vi "Main.vi"() -> ()   [LabVIEW 2012]
uses:
  TypeDefs/States.ctl
  <vilib>/Analysis/NI_AALBase.lvlib
  <vilib>/Analysis/1siggen.llb/Ramp Pattern by Samples.vi
  <vilib>/DAQmx/write.llb/DAQmx Write (Digital Bool 1Line 1Point).vi
  <vilib>/DAQmx/write.llb/DAQmx Write (Analog 1D DBL NChan 1Samp).vi
  <vilib>/DAQmx/read.llb/DAQmx Read (Analog DBL 1Chan 1Samp).vi
  <vilib>/DAQmx/create/channels.llb/DAQmx Create Channel (DO-Digital Output).vi
  <vilib>/DAQmx/create/channels.llb/DAQmx Create Channel (AI-Voltage-Basic).vi
  <vilib>/DAQmx/create/channels.llb/DAQmx Create Channel (AO-Voltage-Basic).vi
  Controls/DAQ Channels.ctl
panel:
  out "Intensity Graph":dbl[][](graph)
  in  "DAQ Channels":T1
  in  "Scan Size":i32
  in  "Start Stop":bool
  in  "stop":bool
  out "Image Viewer":dbl[][](graph)
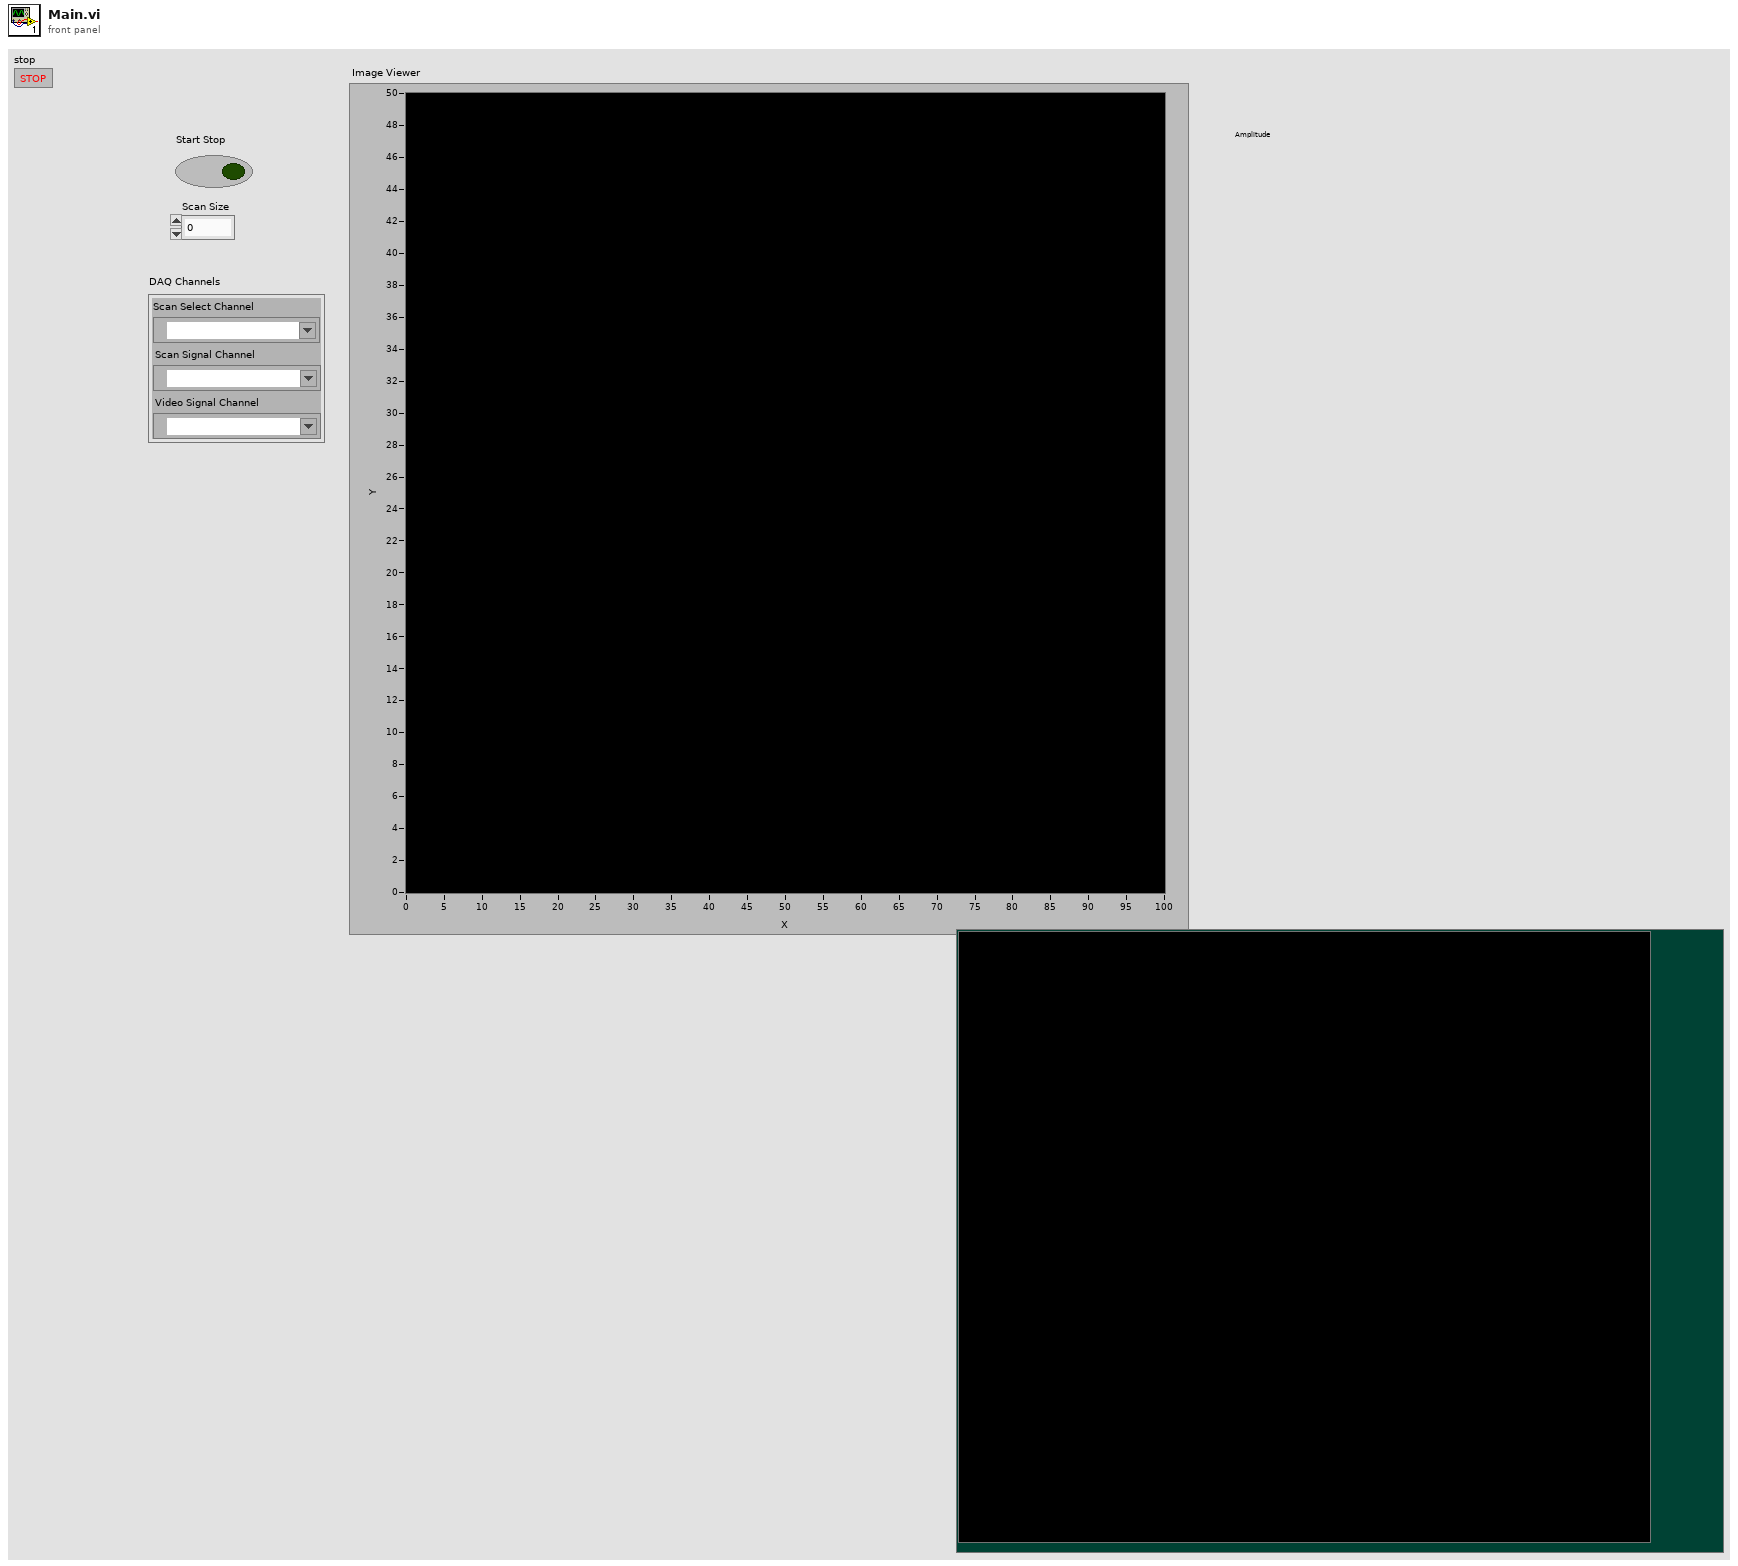
[diagram p1: front panel]
types:
  T1 = typedef "DAQ Channels.ctl" = cluster{"Scan Select Channel":tag, "Scan Signal Channel":tag, "Video Signal Channel":tag}
  T2 = typedef "States.ctl" = enum16{"Standby", "Initialize", "DAQ SetUp", "Run", "Display", "DAQ Clear", "Shut Down", "Exit"}
  T3 = cluster{"task out":refnum<k21>, "task out":refnum<k21>, "task out":refnum<k21>}
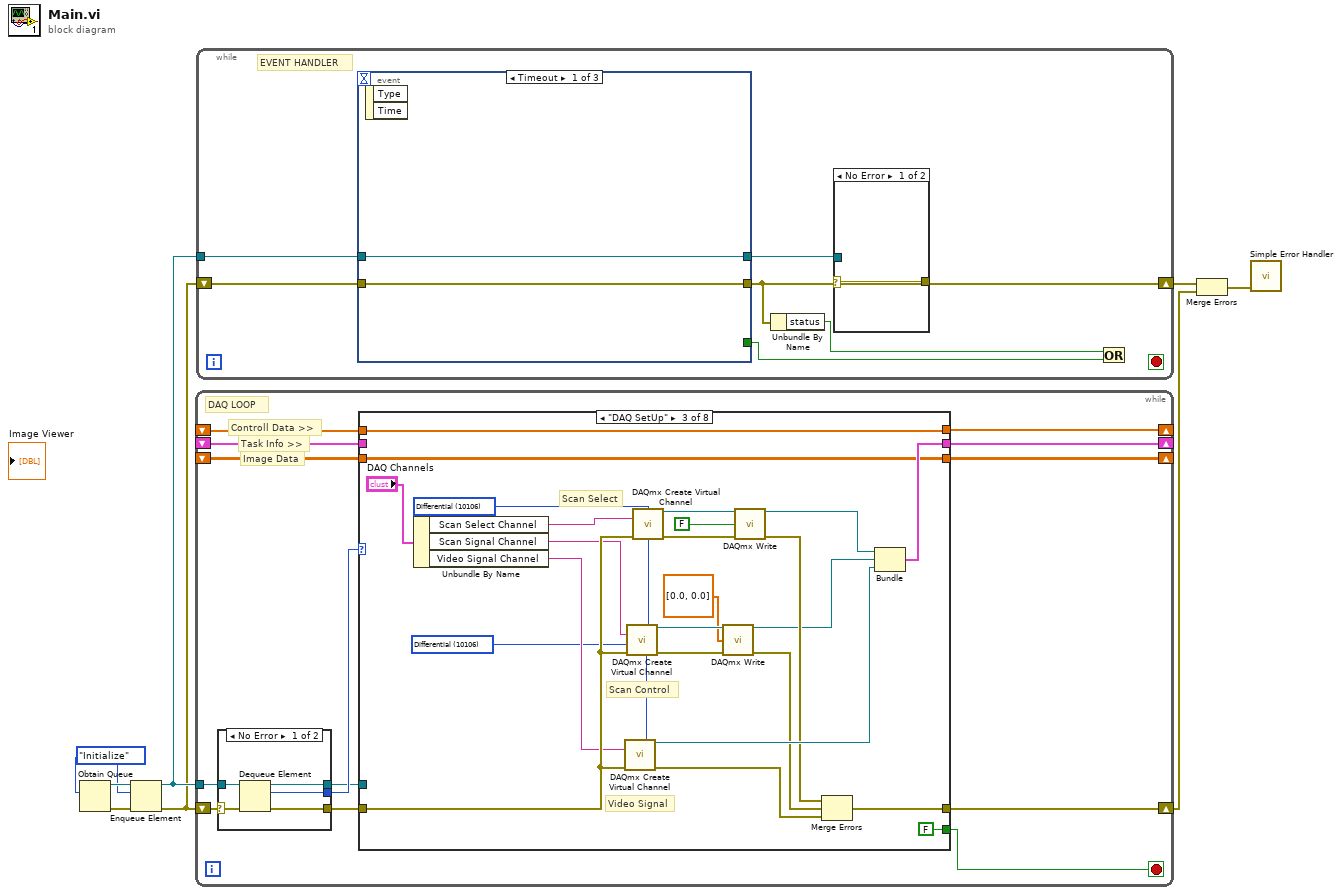
[diagram p0: block diagram]
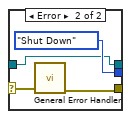
[diagram p2: hidden frame]
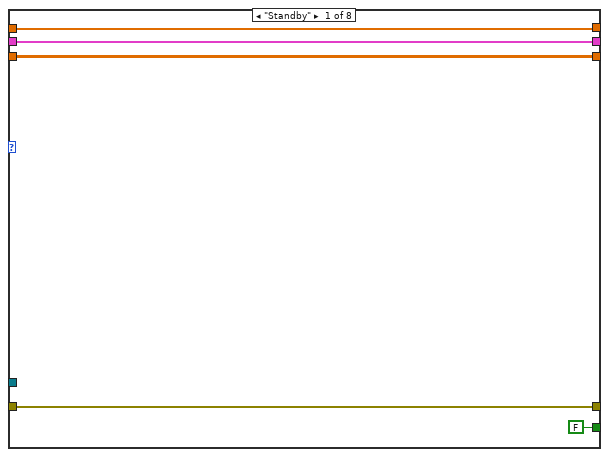
[diagram p3: hidden frame]
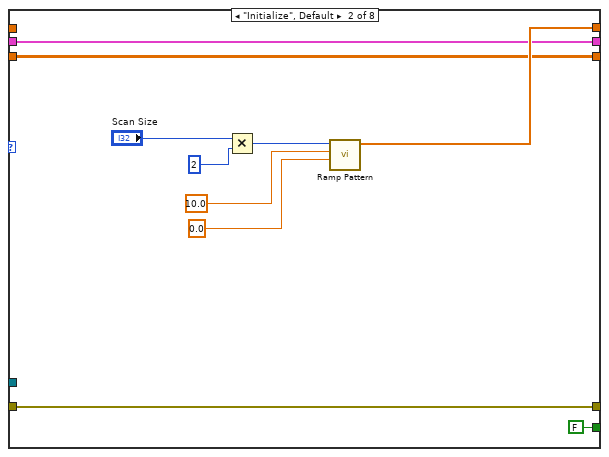
[diagram p4: hidden frame]
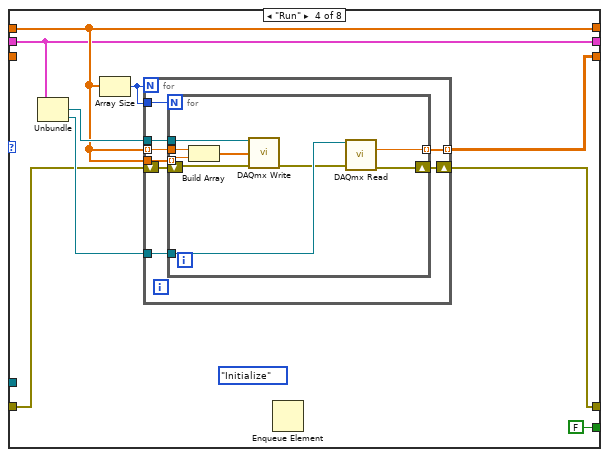
[diagram p5: hidden frame]
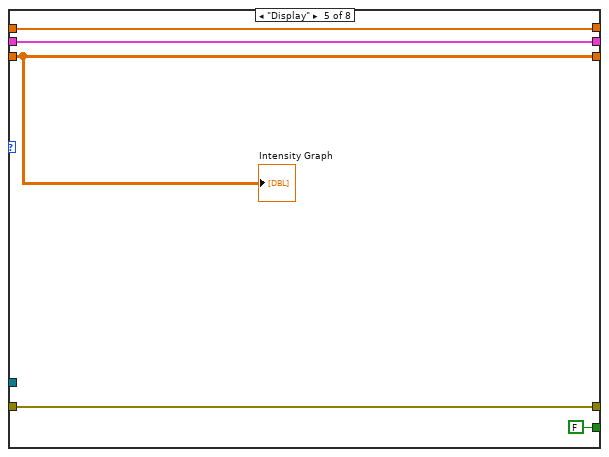
[diagram p6: hidden frame]
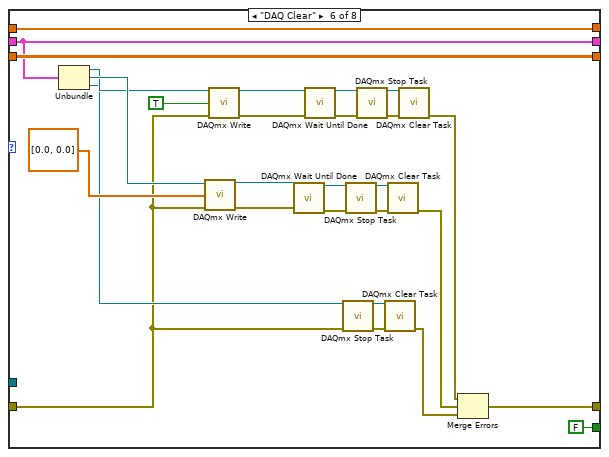
[diagram p7: hidden frame]
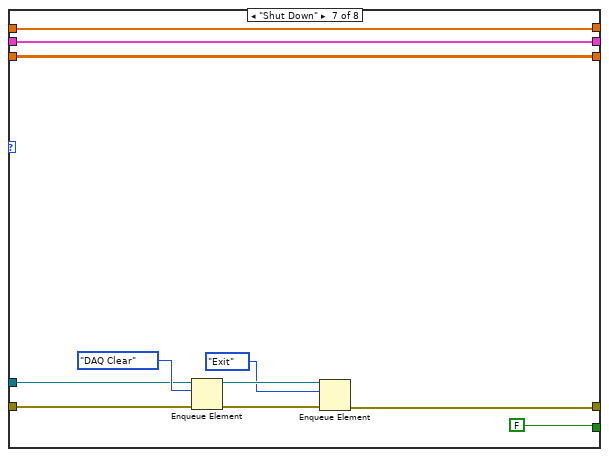
[diagram p8: hidden frame]
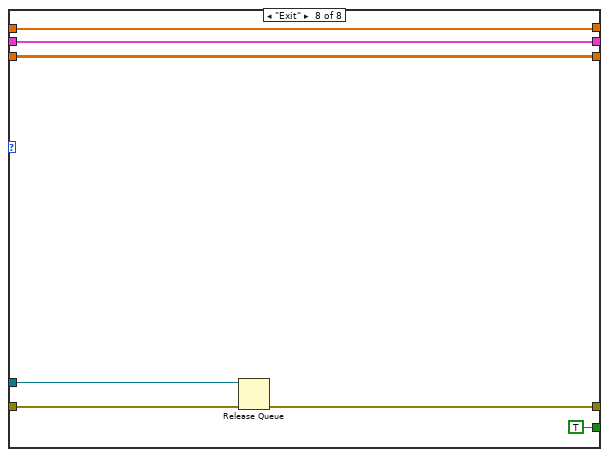
[diagram p9: hidden frame]
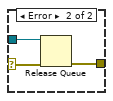
[diagram p10: hidden frame]
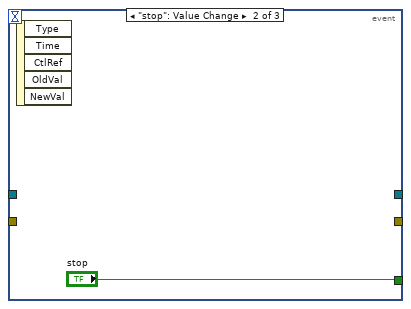
[diagram p11: hidden frame]
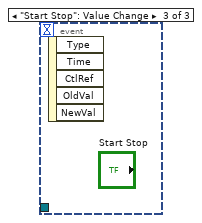
[diagram p12: hidden frame]
diagram:
  w4 = States."Initialize" ("States")
  n1 = Obtain Queue(element data type=w4) -> (queue out=w7:refnum<queue>, error out=w8:errorcluster)  [unwired: 4 in, 1 out]
  n2 = Enqueue Element(queue=w7, element=w4, error in (no error)=w8) -> (queue out=w6:refnum<queue>, error out=w5:errorcluster)  [unwired: 1 in, 1 out]
  n3 = while {
    tunnel: w6 -> [w20]
    shift-right: [w16] -> w1
    shift-left: w5 -> [w21]
    shift-right: [w15] -> _
    shift-left: _ -> [w11]
    shift-right: [w14] -> _
    shift-left: _ -> [w13]
    shift-right: [w12] -> _
    shift-left: _ -> [w10]
    stop <- w9 stop-if-true
    # "Image Data"
    # "Task Info >>"
    # "Controll Data >>"
    # "DAQ LOOP"
    n4 = case shown="No Error" w21 {
      selector: w21 -> [w26 w30]
      tunnel: w20 -> [w25 w27]
      tunnel: [w24 States."Shut Down" ("States")] -> w19
      tunnel: [w23 w27] -> w17
      tunnel: [w22 w29] -> w18
      frame No Error {
        n5 = Dequeue Element(queue=w25, error in (no error)=w26) -> (queue out=w23:refnum<queue>, element=w24:T2, error out=w22:errorcluster)  [unwired: 1 in, 1 out]
      }
      frame Error {
        n6 = call <vilib>:"General Error Handler.vi"("error in (no error)"=w30) -> ("error out"=w29:errorcluster)  [unwired: 10 in, 4 out]
      }
    }
    n7 = case shown="\"DAQ SetUp\"" w19 {
      tunnel: w18 -> [w34 w45 w68 w76 w100 w109 w137 w145]
      tunnel: w17 -> [_ _ _ _ _ _ w136 w144]
      tunnel: [w34 w45 w67 w73 w100 w108 w132 w143] -> w16
      tunnel: [w31 w39 w47 w71 w98 w103 w129 w140] -> w15
      tunnel: [w32 w36 w65 w70 w97 w101 w130 w141] -> w14
      tunnel: w13 -> [w32 w36 _ w70 w97 w101 w130 w141]
      tunnel: w11 -> [w31 _ w47 w71 w98 w103 w129 w140]
      tunnel: [w33 w37 w46 w75 w96 w102 w131 w142] -> w12
      tunnel: w10 -> [w33 w37 w46 _ w96 w102 w131 w142]
      tunnel: [FALSE FALSE FALSE FALSE FALSE FALSE FALSE TRUE] -> w9
      frame "Standby" {
      }
      frame "Initialize", Default {
        n8 = Multiply(x="Scan Size", y=2) -> (x*y=w42:i32)
        n9 = call-poly <vilib>:"Ramp Pattern.vi"("start"=0.0, "end"=10.0, "samples"=w42) -> ("Ramp Pattern"=w39:dbl[])  [unwired: 7 in, 1 out]
      }
      frame "DAQ SetUp" {
        w49 = 10106 items=["Default"=-1, "RSE"=10083, "Differential"=10106, "Pseudodifferential"=12529] ("output terminal configuration")
        w50 = 10106 items=["default"=-1, "RSE"=10083, "NRSE"=10078, "Differential"=10106, "Pseudodifferential"=12529] ("input terminal configuration")
        # "Scan Select"
        # "Scan Control"
        # "Video Signal"
        n10 = Unbundle By Name("DAQ Channels") -> ("Scan Select Channel"=w58:tag, "Scan Signal Channel"=w57:tag, "Video Signal Channel"=w56:tag)
        n11 = call-poly <vilib>:"DAQmx Create Virtual Channel.vi"("input terminal configuration"=w50, "physical channels"=w56, "error in"=w68) -> ("task out"=w66:refnum<k21>, "error out"=w69:errorcluster)  [unwired: 11 in]
        n12 = call-poly <vilib>:"DAQmx Create Virtual Channel.vi"("output terminal configuration"=w49, "physical channels"=w57, "error in"=w68) -> ("task out"=w55:refnum<k21>, "error out"=w54:errorcluster)  [unwired: 11 in]
        n13 = call-poly <vilib>:"DAQmx Create Virtual Channel.vi"("lines"=w58, "error in"=w68) -> ("task out"=w63:refnum<k21>, "error out"=w64:errorcluster)  [unwired: 12 in]
        n14 = call-poly <vilib>:"DAQmx Write.vi"("task/channels in"=w55, "data"=dbl[] [0.0, 0.0], "error in"=w54) -> ("task out"=w52:refnum<k21>, "error out"=w51:errorcluster)  [unwired: 10 in, 1 out]
        n15 = call-poly <vilib>:"DAQmx Write.vi"("task/channels in"=w63, "data"=FALSE, "error in"=w64) -> ("task out"=w60:refnum<k21>, "error out"=w61:errorcluster)  [unwired: 10 in, 1 out]
        n16 = Merge Errors(w61, w51, w69) -> (w67:errorcluster)
        n17 = Bundle("task out"=w60, "task out"=w52, "task out"=w66) -> (w65:T3)  [unwired: 1 in]
      }
      frame "Run" {
        (unwired) States."Initialize" ("States")
        n18 = Unbundle(w70) -> ("task out"=w77:refnum<k21>, "task out"=w78:refnum<k21>)  [unwired: 1 out]
        n19 = Array Size(array=w71) -> (size(s)=w74:i32)
        n20 = for {
          N: w74 -> [_]
          tunnel: w71 -> [w84] mode=indexing
          tunnel: w71 -> [w86]
          tunnel: w78 -> [w85]
          tunnel: w77 -> [w82]
          tunnel: [w81] -> w75 mode=indexing
          tunnel: w74 -> [w80]
          shift-right: [w79] -> w73
          shift-left: w76 -> [w83]
          n21 = for {
            N: w80 -> [_]
            tunnel: w86 -> [w94] mode=indexing
            tunnel: w85 -> [w90]
            tunnel: w84 -> [w95]
            tunnel: w82 -> [w91]
            tunnel: [w88] -> w81 mode=indexing
            shift-right: [w87] -> w79
            shift-left: w83 -> [w92]
            n22 = Build Array(w95, w94) -> (w93:dbl[])
            n23 = call-poly <vilib>:"DAQmx Write.vi"("task/channels in"=w91, "data"=w93, "error in"=w92) -> ("error out"=w89:errorcluster)  [unwired: 10 in, 2 out]
            n24 = call-poly <vilib>:"DAQmx Read.vi"("task/channels in"=w90, "error in"=w89) -> ("data"=w88:dbl, "error out"=w87:errorcluster)  [unwired: 11 in, 1 out]
          }
        }
        n25 = Enqueue Element() -> ()  [unwired: 4 in, 3 out]
      }
      frame "Display" {
        "Intensity Graph" <- w96
      }
      frame "DAQ Clear" {
        n26 = Unbundle(w101) -> ("task out"=w117:refnum<k21>, "task out"=w128:refnum<k21>, "task out"=w110:refnum<k21>)
        n27 = call-poly <vilib>:"DAQmx Write.vi"("task/channels in"=w128, "data"=dbl[] [0.0, 0.0], "error in"=w109) -> ("task out"=w119:refnum<k21>, "error out"=w118:errorcluster)  [unwired: 10 in, 1 out]
        n28 = call-poly <vilib>:"DAQmx Write.vi"("task/channels in"=w117, "data"=TRUE, "error in"=w109) -> ("task out"=w116:refnum<k21>, "error out"=w115:errorcluster)  [unwired: 10 in, 1 out]
        n29 = call <vilib>:"DAQmx Wait Until Done.vi"("task/channels in"=w119, "error in"=w118) -> ("task out"=w123:refnum<k21>, "error out"=w122:errorcluster)  [unwired: 12 in]
        n30 = call <vilib>:"DAQmx Wait Until Done.vi"("task/channels in"=w116, "error in"=w115) -> ("task out"=w127:refnum<k21>, "error out"=w126:errorcluster)  [unwired: 12 in]
        n31 = call <vilib>:"DAQmx Stop Task.vi"("task/channels in"=w110, "error in"=w109) -> ("task out"=w112:refnum<k21>, "error out"=w111:errorcluster)  [unwired: 12 in]
        n32 = call <vilib>:"DAQmx Stop Task.vi"("task/channels in"=w123, "error in"=w122) -> ("task out"=w121:refnum<k21>, "error out"=w120:errorcluster)  [unwired: 12 in]
        n33 = call <vilib>:"DAQmx Stop Task.vi"("task/channels in"=w127, "error in"=w126) -> ("task out"=w125:refnum<k21>, "error out"=w124:errorcluster)  [unwired: 12 in]
        n34 = call <vilib>:"DAQmx Clear Task.vi"("task in"=w112, "error in"=w111) -> ("error out"=w107:errorcluster)  [unwired: 13 in]
        n35 = call <vilib>:"DAQmx Clear Task.vi"("task in"=w121, "error in"=w120) -> ("error out"=w106:errorcluster)  [unwired: 13 in]
        n36 = call <vilib>:"DAQmx Clear Task.vi"("task in"=w125, "error in"=w124) -> ("error out"=w105:errorcluster)  [unwired: 13 in]
        n37 = Merge Errors(w105, w106, w107) -> (w108:errorcluster)
      }
      frame "Shut Down" {
        n38 = Enqueue Element(queue=w136, element=States."DAQ Clear" ("States"), error in (no error)=w137) -> (queue out=w135:refnum<queue>, error out=w134:errorcluster)  [unwired: 1 in, 1 out]
        n39 = Enqueue Element(queue=w135, element=States."Exit" ("States"), error in (no error)=w134) -> (error out=w132:errorcluster)  [unwired: 1 in, 2 out]
      }
      frame "Exit" {
        n40 = Release Queue(queue=w144, error in (no error)=w145) -> (error out=w143:errorcluster)  [unwired: 1 in, 2 out]
      }
    }
  }
  n41 = while {
    tunnel: w6 -> [w151]
    shift-right: [w149] -> w2
    shift-left: w5 -> [w152]
    stop <- _ stop-if-true
    # "EVENT HANDLER"
    n42 = event shown="[0] Timeout" {
      selector: _ -> [_ _ _]
      dyn-events: _ -> [_ _ _]
      timeout: _ -> [_ _ _]
      tunnel: w152 -> [w158 _ _]
      tunnel: [w158 _ _] -> w149
      tunnel: w151 -> [w157 _ _]
      tunnel: [w157 _ _] -> w150
      tunnel: [_ "stop" _] -> w147
      event Timeout {
        n43 = event-data() -> ()  [unwired: 1 in, 2 out]
      }
      event "stop": Value Change {
        n44 = event-data() -> ()  [unwired: 1 in, 5 out]
      }
      event "Start Stop": Value Change {
        n45 = event-data() -> ()  [unwired: 1 in, 5 out]
      }
    }
    n46 = Unbundle By Name(w149) -> ("status"=w148:bool)
    n47 = case shown="No Error" {
      selector: _ -> [w153 w154]
      tunnel: [w153 w156] -> _
      tunnel: w150 -> [_ w155]
      frame No Error {
      }
      frame Error {
        n48 = Release Queue(queue=w155, error in (no error)=w154) -> (error out=w156:errorcluster)  [unwired: 1 in, 2 out]
      }
    }
    n49 = Or(x=w148, y=w147) -> ()  [unwired: 1 out]
  }
  n50 = Merge Errors(w2, w1) -> (w3:errorcluster)
  n51 = call <vilib>:"Simple Error Handler.vi"("error in (no error)"=w3) -> ()  [unwired: 4 in, 5 out]
